vi "AddAxis.vi"(6 "Units":string, 8 "error in (no error)":errorcluster, 9 "Encoder Resolution":string, 10 "Axis Letter":string, 11 "Controller.LV in":refnum<class "Controller.LV.lvclass">) -> (0 "error out":errorcluster, 3 "Controller.LV out":refnum<class "Controller.LV.lvclass">)   [LabVIEW 2019, in "Controller.LV.lvclass"]
uses:
  Controller.LV.lvclass
  Controller.LV.lvclass/Controller.LV.ctl
  drivers/Class/Controller/Controller.lvclass
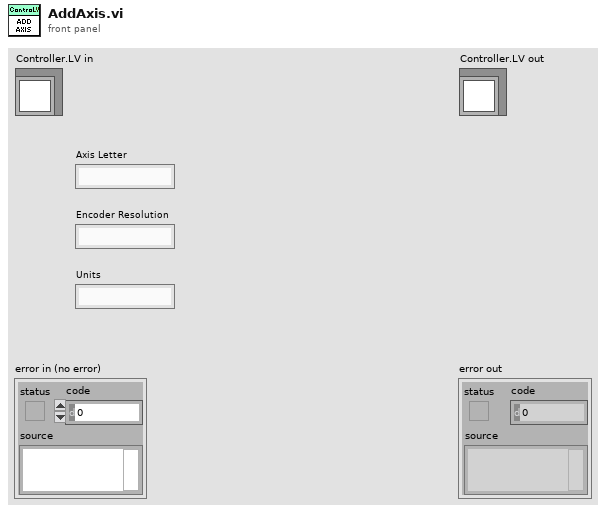
[diagram p1: front panel]
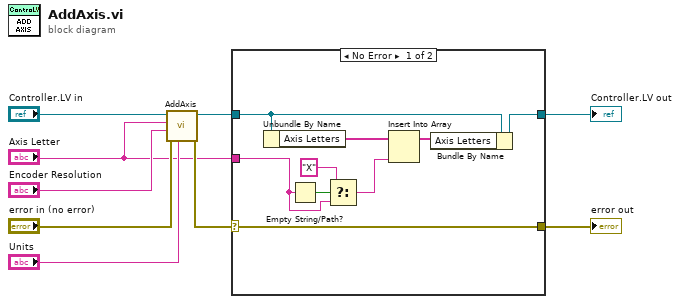
[diagram p0: block diagram]
diagram:
  n1 = call-parent "AddAxis.vi"("Units"="Units", "error in (no error)"="error in (no error)", "Encoder Resolution"="Encoder Resolution", "Axis Letter"="Axis Letter", "Controller in"="Controller.LV in") -> ("error out"=w3:errorcluster, "Controller out"=w7:refnum<class "Controller.LV.lvclass">)  [unwired: 5 in]
  n2 = case shown="No Error" w3 {
    selector: w3 -> [w14 w20]
    tunnel: w7 -> [w16 w19]
    tunnel: [w15 w19] -> w6
    tunnel: "Axis Letter" -> [w11 _]
    tunnel: [w14 w20] -> w5
    frame No Error {
      n3 = Unbundle By Name(w16) -> ("Axis Letters"=w18:string[])
      n4 = Empty String/Path?(string/path=w11) -> (empty?=w13:bool)
      n5 = Select(t="X", s=w13, f=w11) -> (s? t:f=w10:string)
      n6 = Insert Into Array(array=w18, new element=w10) -> (w17:string[])  [unwired: 1 in]
      n7 = Bundle By Name(cluster=w16, "Axis Letters"=w17) -> (w15:refnum<class "Controller.LV.lvclass">)
    }
    frame Error {
    }
  }
  "error out" <- w5
  "Controller.LV out" <- w6
